vi "BelongsToClosedSet.vi"(9 "neighbour":T1, 10 "ClosedSet in":dbl[][](array[numeric])) -> (2 "belongs_to_closedSet":bool)   [LabVIEW 2016]
uses:
  elementGrid.ctl
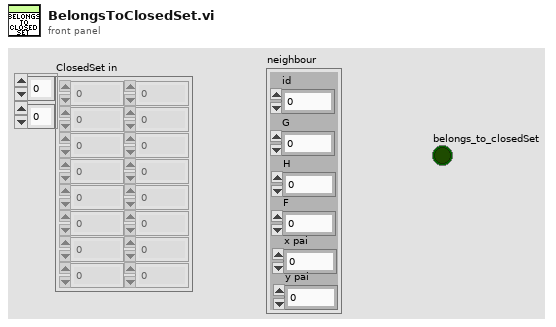
[diagram p1: front panel]
types:
  T1 = typedef "elementGrid.ctl" = cluster{"id":dbl, "G":dbl, "H":dbl, "F":dbl, "x pai":dbl, "y pai":dbl}
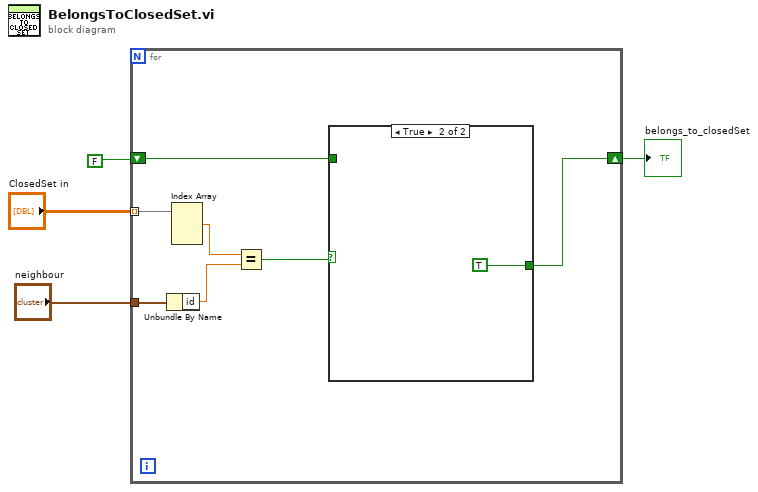
[diagram p0: block diagram]
diagram:
  n1 = for {
    tunnel: "ClosedSet in" -> [w11] mode=indexing
    tunnel: "neighbour" -> [w10]
    shift-right: [w6] -> w1
    shift-left: FALSE -> [w5]
    n2 = Unbundle By Name(w10) -> ("id"=w8:dbl)
    n3 = Index Array(array=w11) -> (element #1=w9:dbl)  [unwired: 3 in, 2 out]
    n4 = Equal?(x=w9, y=w8) -> (x = y?=w7:bool)
    n5 = case shown="True" w7 {
      tunnel: [w12 TRUE] -> w6
      tunnel: w5 -> [w12 _]
      frame False {
      }
      frame True {
      }
    }
  }
  "belongs_to_closedSet" <- w1
